vi "DOE Spare Data.vi"(6 "Data Logger Type":T1=enum."Agilent", 8 "Error In":errorcluster, 10 "Output Array":dbl[](array[numeric]), 11 "Kitchen Cluster in":T2) -> (0 "Error Out":errorcluster, 3 "Kitchen Cluster out 2":T2, 4 "sorted array":i32[](array[numeric]))   [LabVIEW 2020]
uses:
  Type Definitions/DOE Kitchen Control.ctl
  Type Definitions/DOE Data Logger Type.ctl
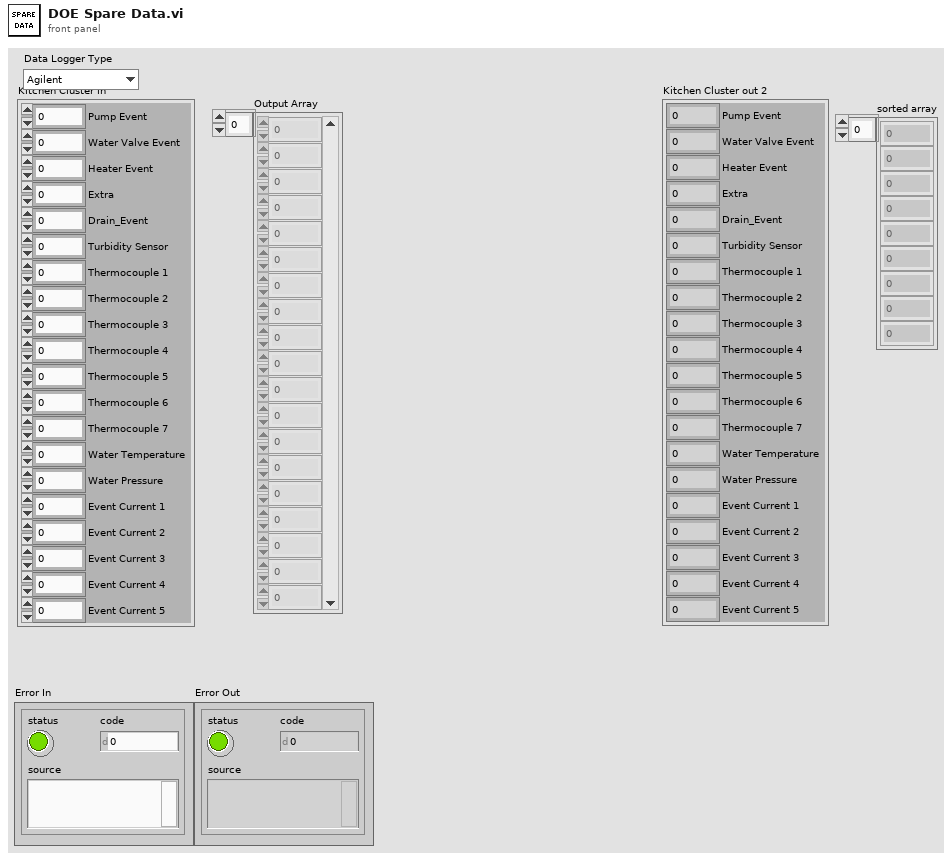
[diagram p1: front panel]
types:
  T1 = typedef "DOE Data Logger Type.ctl" = enum16{"MW100", "Agilent", "Agilent_Laurel_DC_Clamp"}
  T2 = typedef "DOE Kitchen Control.ctl" = cluster{"Drain_Event":i16, "Pump Event":i16, "Water Valve Event":i16, "Heater Event":i16, "Extra":i16, "Turbidity Sensor":dbl, "Thermocouple 1":dbl, "Thermocouple 2":dbl, "Thermocouple 3":dbl, "Thermocouple 4":dbl, "Thermocouple 5":dbl, "Thermocouple 6":dbl, "Water Temperature":dbl, "Water Pressure":dbl, "Event Current 1":dbl, "Event Current 2":dbl, "Event Current 3":dbl, "Event Current 4":dbl, "Event Current 5":dbl, "Thermocouple 7":dbl}
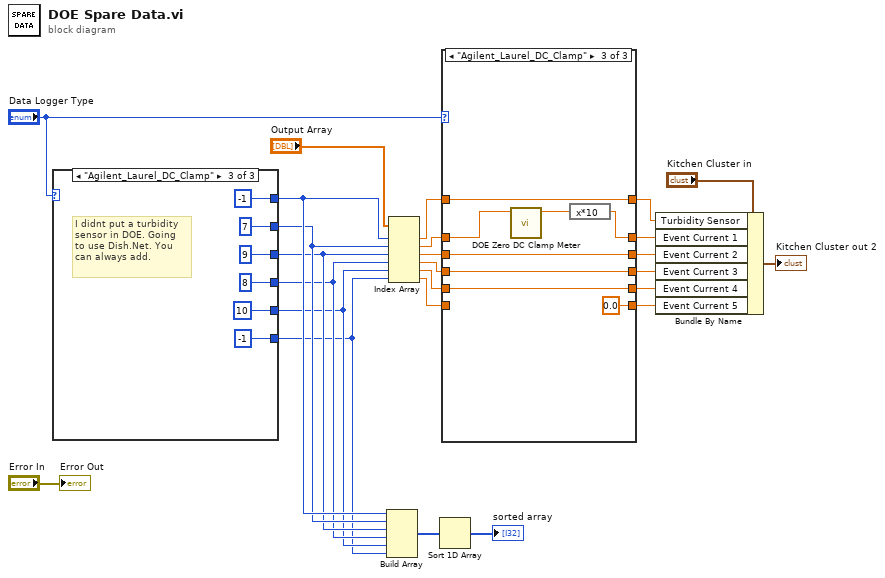
[diagram p0: block diagram]
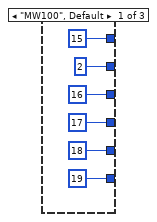
[diagram p4: hidden frame]
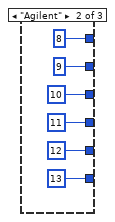
[diagram p5: hidden frame]
diagram:
  n1 = case shown="\"Agilent_Laurel_DC_Clamp\"" "Data Logger Type" {
    tunnel: [19 ("index") 13 ("index") -1 ("index")] -> w16
    tunnel: [18 ("index") 12 ("index") 10 ("index")] -> w17
    tunnel: [17 ("index") 11 ("index") 8 ("index")] -> w18
    tunnel: [16 ("index") 10 ("index") 9 ("index")] -> w19
    tunnel: [2 ("index") 9 ("index") 7 ("index")] -> w20
    tunnel: [15 ("index") 8 ("index") -1 ("index")] -> w21
    frame "MW100", Default {
    }
    frame "Agilent" {
    }
    frame "Agilent_Laurel_DC_Clamp" {
      # "I didnt put a turbidity \nsensor in DOE. Going \nto use Dish.Net. You\ncan always add."
    }
  }
  n2 = Build Array(w21, w20, w19, w18, w17, w16) -> (w15:i32[])
  n3 = Index Array(array="Output Array", index #1=w21, index #2=w20, index #3=w19, index #4=w18, index #5=w17, index #6=w16) -> (element #1=w2:dbl, element #2=w8:dbl, element #3=w7:dbl, element #4=w6:dbl, element #5=w5:dbl, element #6=w4:dbl)
  n4 = Sort 1D Array(array=w15) -> (sorted array=→"sorted array":i32[])
  n5 = case shown="\"Agilent_Laurel_DC_Clamp\"" "Data Logger Type" {
    tunnel: [w44 w50 0.0 ("Numeric")] -> w13
    tunnel: [w45 w51 w57] -> w12
    tunnel: [w46 w52 w58] -> w11
    tunnel: [w47 w53 w59] -> w10
    tunnel: [w48 w54 w63] -> w9
    tunnel: w8 -> [w48 w54 w62]
    tunnel: w7 -> [w47 w53 w59]
    tunnel: w6 -> [w46 w52 w58]
    tunnel: w5 -> [w45 w51 w57]
    tunnel: w4 -> [w44 w50 _]
    tunnel: w2 -> [w49 w55 w60]
    tunnel: [w49 w55 w60] -> w1
    frame "MW100", Default {
    }
    frame "Agilent" {
    }
    frame "Agilent_Laurel_DC_Clamp" {
      n6 = call "DOE Zero DC Clamp Meter.vi"("Uncorrected Voltage"=w62) -> ("Corrected Voltage"=w61:dbl)  [unwired: 10 in]
      n7 = expression code="x*10"(w61) -> (w63:dbl)
    }
  }
  n8 = Bundle By Name(cluster="Kitchen Cluster in", "Turbidity Sensor"=w1, "Event Current 1"=w9, "Event Current 2"=w10, "Event Current 3"=w11, "Event Current 4"=w12, "Event Current 5"=w13) -> (→"Kitchen Cluster out 2":T2)
  "Error Out" <- "Error In"
